vi "Coordinate from AFM to inkscape.vi"() -> ()   [LabVIEW 2013]
panel:
  out "inkscape information":T1
  in  "AFM information":T1
  in  "Global offset":cluster{"x":dbl, "y":dbl}
  # "20-40umxoffset"
  # "20-40umyoffset"
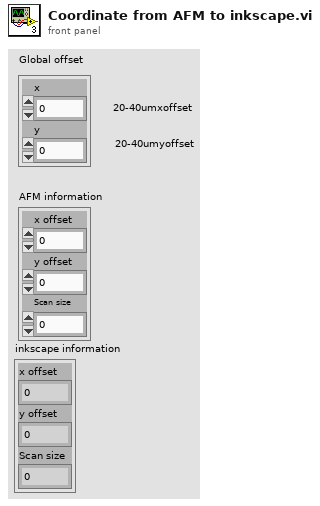
[diagram p1: front panel]
types:
  T1 = cluster{"x offset":dbl, "y offset":dbl, "Scan size":dbl}
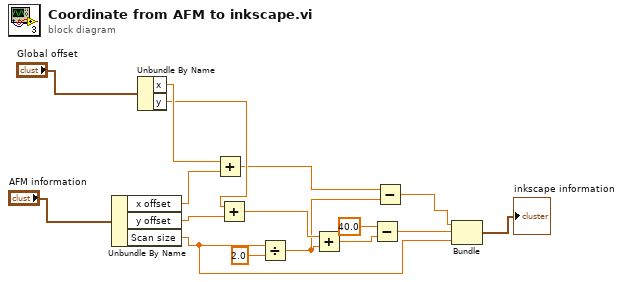
[diagram p0: block diagram]
diagram:
  n1 = Unbundle By Name("AFM information") -> ("x offset"=w13:dbl, "y offset"=w11:dbl, "Scan size"=w2:dbl)
  n2 = Unbundle By Name("Global offset") -> ("x"=w14:dbl, "y"=w12:dbl)
  n3 = Add(x=w14, y=w13) -> (x+y=w9:dbl)
  n4 = Add(x=w12, y=w11) -> (x+y=w8:dbl)
  n5 = Divide(x=w2, y=2.0) -> (x/y=w7:dbl)
  n6 = Add(x=w8, y=w7) -> (x+y=w5:dbl)
  n7 = Subtract(x=40.0, y=w5) -> (x-y=w3:dbl)
  n8 = Subtract(x=w9, y=w7) -> (x-y=w4:dbl)
  n9 = Bundle(w4, w3, "Scan size"=w2) -> (→"inkscape information":cluster{dbl, dbl, "Scan size":dbl})  [unwired: 1 in]
